vi "GetDefaultParams.vi"(8 "error in (no error)":errorcluster, 11 "PathToIni":path) -> (0 "error out":errorcluster, 2 "clConfig":T1, 3 "PathToClass":path)   [LabVIEW 2014, in "AnalysisPlugins.lvlib" / "AnalysisPluginsBase.lvclass"]
uses:
  AnalysisPluginsBase.lvclass
  FitterBaseClass/Typedefs/clAnalysisConfig.ctl
  <vilib>/Utility/config.llb/Read Key (Path).vi
  <vilib>/Utility/error.llb/Error Cluster From Error Code.vi
  <vilib>/ErrorRing/Error Ring.xnode
  <vilib>/Utility/config.llb/NI_LVConfig.lvlib
  FitterBaseClass/FitterBase.lvclass
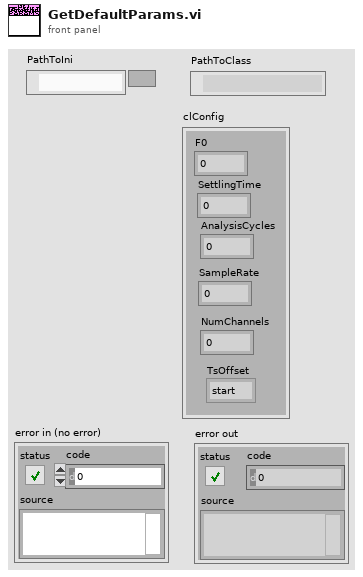
[diagram p1: front panel]
types:
  T1 = typedef "AnalysisPlugins.lvlib/FitterBase.lvclass/clAnalysisConfig.ctl" = cluster{"F0":u32, "SettlingTime":dbl, "AnalysisCycles":dbl, "SampleRate":dbl, "NumChannels":u32, "TsOffset":enum16{"start", "middle", "end"}}
  T2 = typedef "NI_LVConfig.lvlib/Config Data RefNum.ctl" = refnum<k1>
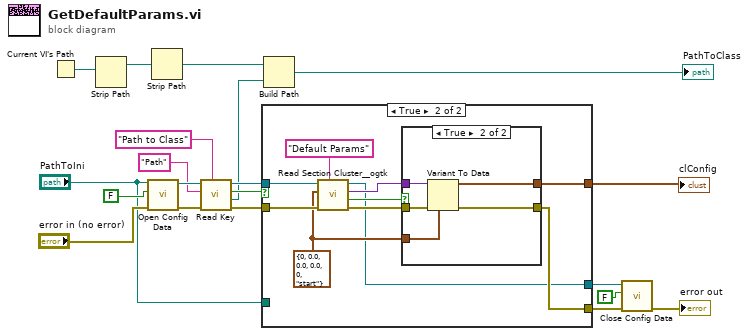
[diagram p0: block diagram]
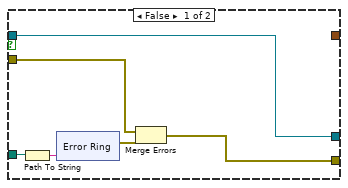
[diagram p2: hidden frame]
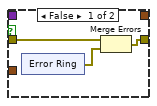
[diagram p3: hidden frame]
diagram:
  n1 = Current VI's Path() -> (path=w5:path)
  n2 = Strip Path(path=w5) -> (stripped path=w4:path)  [unwired: 1 out]
  n3 = call <vilib>:"Open Config Data.vi"("error in (no error)"="error in (no error)", "create file if necessary (T)"=FALSE, "configuration file path"="PathToIni") -> ("error out"=w18:errorcluster, "refnum"=w17:T2)  [unwired: 6 in, 1 out]
  n4 = Strip Path(path=w4) -> (stripped path=w1:path)  [unwired: 1 out]
  n5 = call-poly <vilib>:"Read Key.vi"("section"="Path to Class", "error in (no error)"=w18, "key"="Path", "refnum"=w17) -> ("error out"=w13:errorcluster, "value"=w3:path, "found?"=w11:bool, "refnum out"=w14:T2)  [unwired: 4 in]
  n6 = case shown="True" w11 {
    tunnel: w14 -> [w26 w43]
    tunnel: w13 -> [w22 w42]
    tunnel: [_ w38] -> w12
    tunnel: [w21 w37] -> w10
    tunnel: [w26 w34] -> w7
    tunnel: "PathToIni" -> [w24 _]
    frame False {
      n7 = Path To String(path=w24) -> (string=w25:string)
      n8 = xnode "Error Ring"("parameter 0"=w25) -> ("error out"=w23:errorcluster)
      n9 = Merge Errors(w22, w23) -> (w21:errorcluster)
    }
    frame True {
      w39 = T1 {"F0"=0, "SettlingTime"=0.0, "AnalysisCycles"=0.0, "SampleRate"=0.0, "NumChannels"=0, "TsOffset"=enum."start"} ("clConfig")
      n10 = call <userlib>:"Read Section Cluster__ogtk.vi"("section (optional)"="Default Params", "error in (no error)"=w42, "Section Formatted Cluster Type"=w39, "refnum"=w43) -> ("error out"=w35:errorcluster, "all found?"=w36:bool, "Section Formatted Cluster"=w40:variant, "dup refnum"=w34:T2)  [unwired: 3 in, 1 out]
      n11 = case shown="True" w36 {
        tunnel: w35 -> [w45 w56]
        tunnel: w40 -> [_ w55]
        tunnel: w39 -> [_ w54]
        tunnel: [_ w53] -> w38
        tunnel: [w44 w52] -> w37
        frame False {
          n12 = xnode "Error Ring"() -> ("error out"=w46:errorcluster)
          n13 = Merge Errors(w45, w46) -> (w44:errorcluster)
        }
        frame True {
          n14 = Variant To Data(error in=w56, type=w54, Variant=w55) -> (data=w53:T1, error out=w52:errorcluster)
        }
      }
    }
  }
  "clConfig" <- w12
  n15 = Build Path(base path=w1, name or relative path=w3) -> (appended path=→"PathToClass":path)
  n16 = call <vilib>:"Close Config Data.vi"("error in (no error)"=w10, "write file if changed (T)"=FALSE, "refnum"=w7) -> ("error out"=→"error out":errorcluster)  [unwired: 7 in, 1 out]
